vi "Vision Research Phantom Series PhCon PhGetFrameRateRange.vi"(0 "CN in":u32=1, 2 "Res":cluster{"x":i32, "y":i32}, 5 "Error In (no error)":errorcluster) -> (14 "CN out":u32=1, 16 "pMaxFrameRate(out)":u32, 17 "pMinFrameRate(out)":u32, 19 "Error Out":errorcluster)   [LabVIEW 2013, in "VRI.lvlib"]
uses:
  VRI.lvlib
  Phantom DLLs/PhCon.Dll
panel:
  # "For instructions on the use of this VI, press Ctrl+H to display the help window and move the mouse over the icon, controls, and indicators"
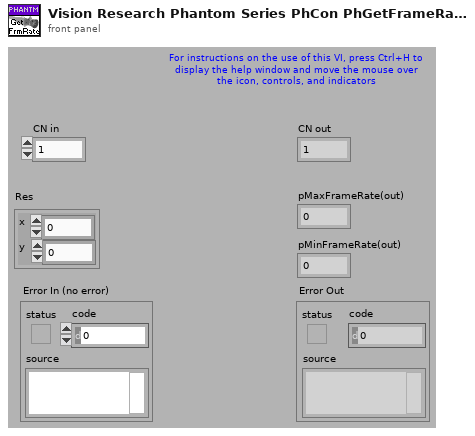
[diagram p1: front panel]
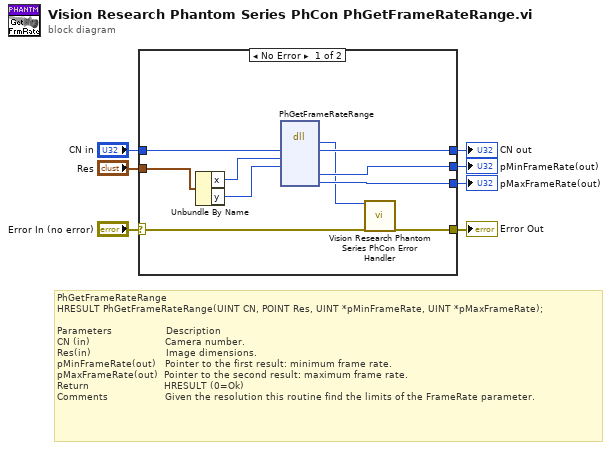
[diagram p0: block diagram]
diagram:
  # "PhGetFrameRateRange\nHRESULT PhGetFrameRateRange(UINT CN, POINT Res, UINT *pMinFrameRate, UINT *pMaxFrameRate);\n\nParameters                  Description\nCN (in)                         Camera number.\nRes(in)                         Image dimensions.\npMinFrameRate(out)   Pointer to the first result: minimum frame rate.\npMaxFrameRate(out)  Pointer to the second result: maximum frame rate.\nReturn                         HRESULT (0=Ok)\nComments                   Given the resolution this routine find the limits of the FrameRate parameter."
  n1 = case shown="No Error" "Error In (no error)" {
    selector: "Error In (no error)" -> [w17 w19]
    tunnel: [w16 w19] -> w6
    tunnel: "CN in" -> [w15 w18]
    tunnel: [w14 w18] -> w4
    tunnel: "Res" -> [w13 _]
    tunnel: [w12 _] -> w2
    tunnel: [w11 _] -> w1
    frame No Error {
      n2 = Unbundle By Name(w13) -> ("x"=w9:i32, "y"=w8:i32)
      n3 = dll-call lib="C:/Projects/SDK/64-bit/Vision Research Phantom Series Labview Driver/Phantom DLLs/PhCon.dll" fn="PhGetFrameRateRange"("CN"=w15, "x"=w9, "y"=w8) -> ("HRESULT"=w10:i32, "CN"=w14:u32, "pMinFrameRate"=w12:u32, "pMaxFrameRate"=w11:u32)  [unwired: 5 in, 4 out]
      n4 = call "Vision Research Phantom Series PhCon Error Handler.vi"("ErrNo"=w10, "Error In (no error)"=w17) -> ("Error Out"=w16:errorcluster)  [unwired: 17 out]
    }
    frame Error {
    }
  }
  "Error Out" <- w6
  "CN out" <- w4
  "pMinFrameRate(out)" <- w2
  "pMaxFrameRate(out)" <- w1
